vi "选中背景色.vi"(8 "错误输入（无错误）":errorcluster, 11 "引用":refnum<k24>) -> (0 "错误输出":errorcluster, 3 "引用输出":refnum<k24>)   [LabVIEW 2020]
uses:
  D:/SuperPython-master/ScintillaNET.dll
  ScintillaNET.dll
  System.Drawing
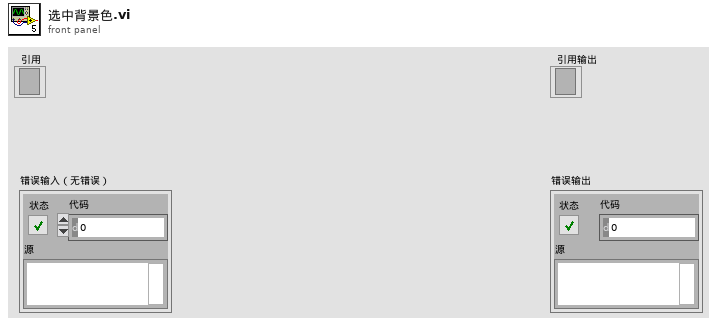
[diagram p1: front panel]
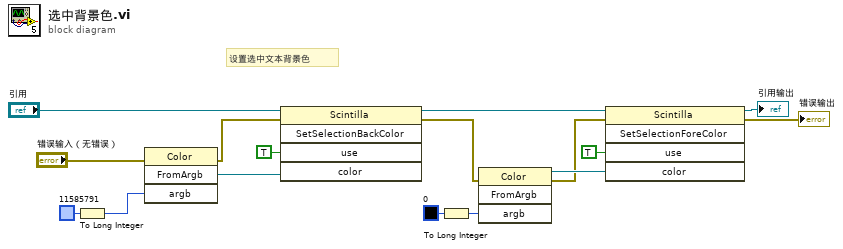
[diagram p0: block diagram]
diagram:
  # "设置选中文本背景色"
  n1 = To Long Integer(number=u32 11585791) -> (32bit integer=w14:i32)
  n2 = invoke class="Color" method="FromArgb"(error in="错误输入（无错误）", "argb"=w14) -> (error out=w12:errorcluster, "FromArgb"=w10:refnum<k24>)  [unwired: 2 in, 2 out]
  n3 = invoke class="Scintilla" method="SetSelectionBackColor"(reference="引用", error in=w12, "use"=TRUE, "color"=w10) -> (reference out=w5:refnum<k24>, error out=w3:errorcluster)  [unwired: 1 in, 3 out]
  n4 = To Long Integer(number=u32 0) -> (32bit integer=w8:i32)
  n5 = invoke class="Color" method="FromArgb"(error in=w3, "argb"=w8) -> (reference out=w6:refnum<k24>, error out=w4:errorcluster)  [unwired: 2 in, 2 out]
  n6 = invoke class="Scintilla" method="SetSelectionForeColor"(reference=w5, error in=w4, "use"=TRUE, "color"=w6) -> (reference out=→"引用输出":refnum<k24>, error out=→"错误输出":errorcluster)  [unwired: 1 in, 3 out]
